vi "Read-Save DefaultSerialPort.vi"(6 "Task":enum16{"Save", "Read"}(ring)=enum."Read", 10 "steps per degree":dbl=1.67, 11 "VISA":refnum<visa-resource-name>) -> (0 "Pref Path":path, 2 "steps per degree out":dbl=1.67, 3 "VISA out":refnum<visa-resource-name>)   [LabVIEW 2022 SP3]
panel:
  out "text":string
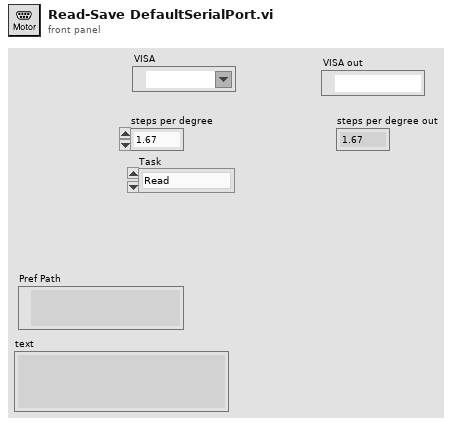
[diagram p1: front panel]
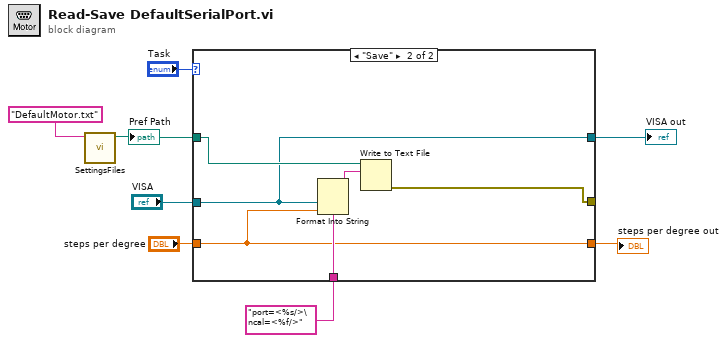
[diagram p0: block diagram]
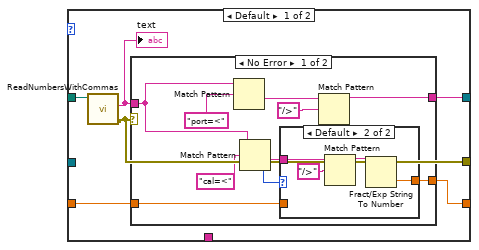
[diagram p2: hidden frame]
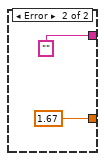
[diagram p4: hidden frame]
diagram:
  n1 = call "SettingsFiles.vi"("settings file name"="DefaultMotor.txt" ("name or relative path")) -> ("file path"=w1:path)  [unwired: 9 in, 1 out]
  "Pref Path" <- w1
  n2 = case shown="\"Save\"" "Task" {
    tunnel: "VISA" -> [_ w34]
    tunnel: w1 -> [w13 w37]
    tunnel: [w11 w35] -> _
    tunnel: [w14 w34] -> w5
    tunnel: "port=<%s/>\ncal=<%f/>" ("format string") -> [_ w33]
    tunnel: "steps per degree" -> [w9 w32]
    tunnel: [w10 w32] -> w3
    frame Default {
      n3 = call "ReadNumbersWithCommas.vi"("file (use dialog)"=w13) -> ("error out"=w11:errorcluster, "text"=w12:string)  [unwired: 7 in, 2 out]
      "text" <- w12
      n4 = case shown="No Error" w11 {
        tunnel: [w22 "" ("Notes")] -> w14
        tunnel: w12 -> [w18 _]
        tunnel: [w17 1.67] -> w10
        tunnel: w9 -> [w15 _]
        frame No Error {
          n5 = Match Pattern(string=w18, regular expression="port=<" ("format string")) -> (after substring=w24:string)  [unwired: 1 in, 3 out]
          n6 = Match Pattern(string=w18, regular expression="cal=<" ("format string")) -> (after substring=w20:string, offset past match=w16:i32)  [unwired: 1 in, 2 out]
          n7 = case shown="Default" w16 {
            tunnel: w20 -> [_ w28]
            tunnel: [w25 w26] -> w17
            tunnel: w15 -> [w25 _]
            frame -1 {
            }
            frame Default {
              n8 = Match Pattern(string=w28, regular expression="/>" ("format string")) -> (before substring=w27:string)  [unwired: 1 in, 3 out]
              n9 = Fract/Exp String To Number(string=w27) -> (number=w26:dbl)  [unwired: 3 in, 1 out]
            }
          }
          n10 = Match Pattern(string=w24, regular expression="/>" ("format string")) -> (before substring=w22:string)  [unwired: 1 in, 3 out]
        }
        frame Error {
        }
      }
    }
    frame "Save" {
      n11 = Format Into String(format string=w33, w34, w32) -> (resulting string=w36:string)  [unwired: 2 in, 1 out]
      n12 = Write to Text File(file (use dialog)=w37, text=w36) -> (error out=w35:errorcluster)  [unwired: 2 in, 2 out]
    }
  }
  "VISA out" <- w5
  "steps per degree out" <- w3
